vi "GVAbschalten.vi"() -> ()   [LabVIEW 2010]
panel:
  in  "NeueMethode":bool
  in  "JetztAbschalten":bool
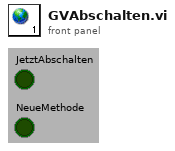
[diagram p1: front panel]
diagram:
